vi "Main.vi"() -> ()   [LabVIEW 2020]
uses:
  Libraries/Adquisition/Adquisition.lvlib
panel:
  out "Data":dbl[](graph)
  in  "Stop":bool
  in  "Start":bool
  in  "Exit":bool
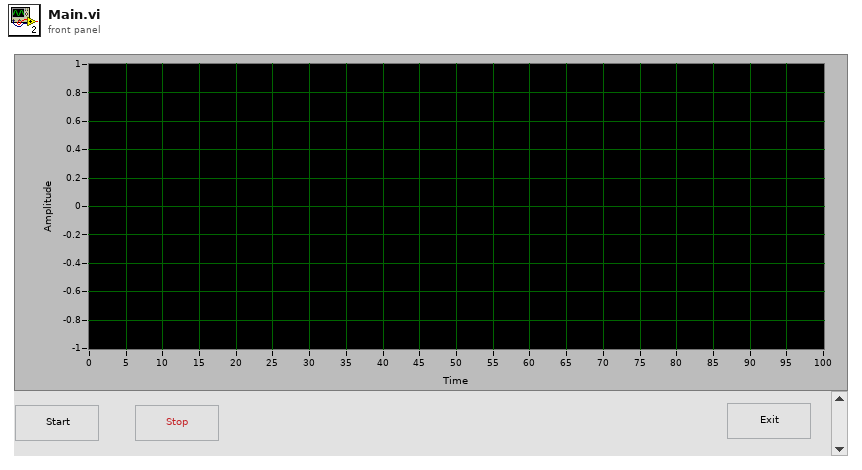
[diagram p1: front panel]
types:
  T1 = typedef "Adquisition.lvlib/Broadcast Events--cluster.ctl" = cluster{"Module Did Init":refnum<user-event>, "Status Updated":refnum<user-event>, "Error Reported":refnum<user-event>, "Module Did Stop":refnum<user-event>, "Update Module Execution Status":refnum<user-event>, "Data Acquired":refnum<user-event>}
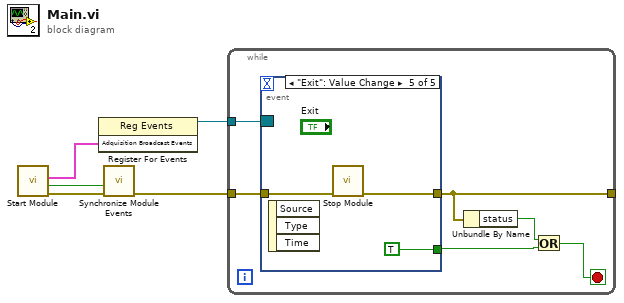
[diagram p0: block diagram]
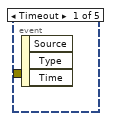
[diagram p2: hidden frame]
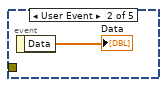
[diagram p3: hidden frame]
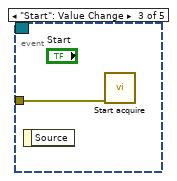
[diagram p4: hidden frame]
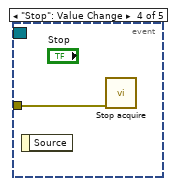
[diagram p5: hidden frame]
diagram:
  n1 = call "Start Module.vi"() -> ("error out"=w5:errorcluster, "Wait for Event Sync?"=w1:bool, "Adquisition Broadcast Events"=w4:T1)  [unwired: 8 in, 1 out]
  n2 = register-events(w4) -> (reference out=w3:refnum<event-registration>)  [unwired: 2 in, 1 out]
  n3 = call "Synchronize Module Events.vi"("error in (no error)"=w5, "Wait for Event Sync?"=w1) -> ("error out"=w2:errorcluster)  [unwired: 9 in]
  n4 = while {
    tunnel: w3 -> [w11]
    tunnel: w2 -> [w10]
    tunnel: [w9] -> _
    stop <- w7 stop-if-true
    n5 = event shown="[4] \"Exit\": Value Change" {
      selector: w11 -> [_ _ _ _ _]
      dyn-events: _ -> [_ _ _ _ _]
      timeout: _ -> [_ _ _ _ _]
      tunnel: w10 -> [_ _ w13 w14 w17]
      tunnel: [_ _ _ _ w16] -> w9
      tunnel: [_ _ _ _ TRUE] -> w6
      event Timeout {
        n6 = event-data() -> ()  [unwired: 1 in, 3 out]
      }
      event User Event {
        n7 = event-data() -> ("Data"=→"Data":dbl[])  [unwired: 1 in]
      }
      event "Start": Value Change {
        n8 = event-data() -> ()  [unwired: 1 in, 1 out]
        n9 = call "Start acquire.vi"("error in (no error)"=w13) -> ()  [unwired: 10 in, 1 out]
      }
      event "Stop": Value Change {
        n10 = event-data() -> ()  [unwired: 1 in, 1 out]
        n11 = call "Stop acquire.vi"("error in (no error)"=w14) -> ()  [unwired: 10 in, 1 out]
      }
      event "Exit": Value Change {
        n12 = event-data() -> ()  [unwired: 1 in, 3 out]
        n13 = call "Stop Module.vi"("error in (no error)"=w17) -> ("error out"=w16:errorcluster)  [unwired: 10 in]
      }
    }
    n14 = Unbundle By Name(w9) -> ("status"=w8:bool)
    n15 = Or(x=w8, y=w6) -> (x .or. y?=w7:bool)
  }
